vi "Assign DIO Bits To Notify Motion Status.vi"(4 "Bit Level (Low)":bool, 5 "error in (no error)":errorcluster, 6 "Bit Number (0)":i32 min=0 max=15, 7 "Axis (1)":i32=1 min=1 max=3, 8 "VISA resource name":refnum<visa-resource-name>) -> (0 "error out":errorcluster, 3 "VISA resource name out":refnum<visa-resource-name>)   [LabVIEW 2018, in "Newport ESP301.lvlib"]
doc: "This command is used to assign DIO bits for notifying the motion status – moving or not moving – of a selected axis. When the selected axis is not moving, the DIO bit state changes to the level specified with this command (refer parameter <B>Bit Level (Low)</B>).\n<B>NOTE</B>: The direction of the DIO port (A, B) the desired bit belongs to, should be set to \"output\" in order for the DIO bit to be set accurately. Refer <B>set DIO port A, B, C direction</B> command for further details.\n<B>NOTE</B>: If a motion feature, such as origin search, involves a sequence of moves, the motion status will be set to not moving only after the entire sequence of moves has completed."
uses:
  Newport ESP301.lvlib
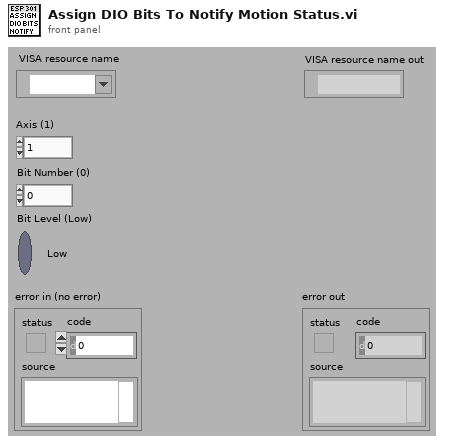
[diagram p1: front panel]
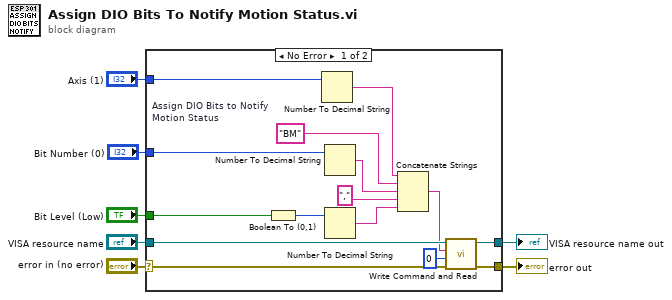
[diagram p0: block diagram]
diagram:
  n1 = case shown="No Error" "error in (no error)" {
    selector: "error in (no error)" -> [w21 w24]
    tunnel: [w20 w24] -> w7
    tunnel: "VISA resource name" -> [w22 w23]
    tunnel: [w19 w23] -> w6
    tunnel: "Axis (1)" -> [w15 _]
    tunnel: "Bit Level (Low)" -> [w13 _]
    tunnel: "Bit Number (0)" -> [w11 _]
    frame No Error {
      w16 = "BM"  # Assign DIO Bits to Notify Motion Status
      n2 = Boolean To (0,1)(Boolean=w13) -> (0, 1=w17:i16)
      n3 = Number To Decimal String(number=w15) -> (decimal integer string=w18:string)  [unwired: 1 out]
      n4 = Number To Decimal String(number=w11) -> (decimal integer string=w10:string)  [unwired: 1 out]
      n5 = Number To Decimal String(number=w17) -> (decimal integer string=w9:string)  [unwired: 1 out]
      n6 = Concatenate Strings(w18, w16, w10, "," ("Assign DIO Bits to Inhibit Motion"), w9) -> (w14:string)
      n7 = call "Write Command and Read.vi"("error in (no error)"=w21, "Bytes to read (100)"=u32 0, "Command"=w14, "VISA resource name"=w22) -> ("error out"=w20:errorcluster, "VISA resource name out"=w19:refnum<visa-resource-name>)  [unwired: 1 in, 3 out]
    }
    frame Error {
    }
  }
  "error out" <- w7
  "VISA resource name out" <- w6
